vi "Autonomous Independent.vi"() -> ()   [LabVIEW 2014]
doc: "This VI is called when autonomous begins, and will automatically be terminated when autonomous ends. You can carry out timed or sensor driven robot movement independently without needing to return to the caller."
uses:
  <vilib>/Rock Robotics/WPI/Solenoid/WPI_SolenoidValue.ctl
  <vilib>/Rock Robotics/WPI/Joystick/WPI_JoystickGetSetRefNum.vi
  <vilib>/Rock Robotics/Network Tables/SD Write Numeric Array.vi
  <vilib>/Rock Robotics/Network Tables/SD Read Boolean.vi
  <vilib>/Rock Robotics/Network Tables/SD Write Boolean.vi
  <vilib>/Rock Robotics/WPI/RobotDrive/WPI_RobotDriveGetSetRefNum.vi
  <vilib>/Rock Robotics/WPI/RobotDrive/WPI_RobotDriveMecanumDrive_Cartesian.vi
  <vilib>/Rock Robotics/WPI/Solenoid/WPI_SolenoidSetEnum.vi
  <vilib>/Rock Robotics/Network Tables/SD Write String.vi
  Robot Global Data.vi
panel:
  out "Mode 3":bool
  out "error out":errorcluster
  out "Mode 1":bool
  out "Mode 0":bool
  in  "Turn":bool=TRUE
  in  "Lift":bool=TRUE
  in  "Move_Forward":bool=TRUE
  in  "Start":bool=TRUE
  in  "Begin":bool=TRUE
  in  "Lift_Time":dbl
  in  "Move_Foward_Time":dbl
  in  "Turn_Time":dbl
  in  "Start_Time":dbl
  # "Be sure to right-click and choose Data Operations>>Make Current Value default if you want to save the array values with the VI"
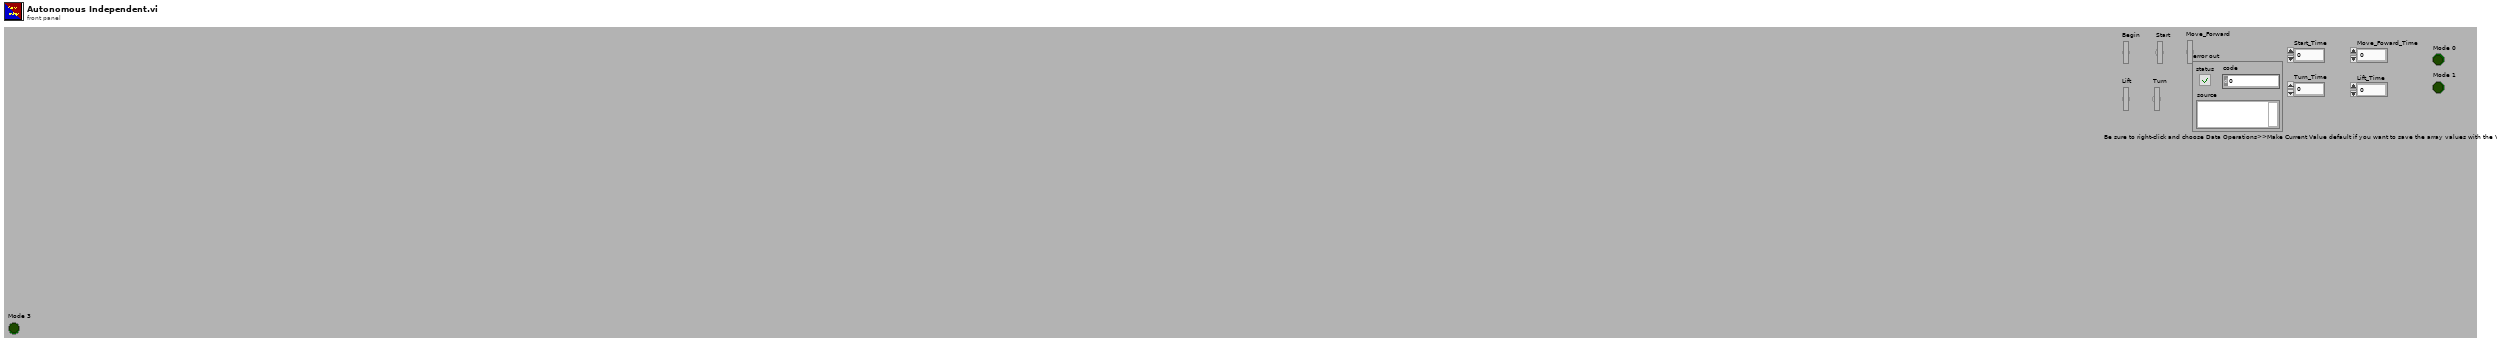
[diagram p1: front panel]
types:
  T1 = typedef "WPI_JoystickDevRef.ctl" = cluster{"Device":T2}
  T2 = typedef "WPI_JoystickDeviceEnum.ctl" = enum16{"USB 0", "USB 1", "USB 2", "USB 3", "USB 4", "USB 5"}
  T3 = typedef "WPI_SolenoidValue.ctl" = enum16{"Off", "On", "Forward", "Reverse"}
  T4 = typedef "WPI_MotorControlDeviceRef.ctl" = cluster{"DeviceStatus":errorcluster, "Type":T5, "PWM":cluster{"Controller":T6, "PWM Channel":T7, "DeadBand":T8}, "CAN":cluster{"Device Number":u8, "Control Mode":T9, "Semaphore":T10, "Max Vout":dbl, "TalonSRX Control Mode":T11}, "Invert":bool, "TransformRef":T12, "InvTransformRef":T12}
  T5 = typedef "WPI_MotorControlType.ctl" = enum16{"PWM", "CAN", "CANTalonSRX"}
  T6 = typedef "FPGA_TypedefDigitalModule.ctl" = enum16{"Controller 1"}
  T7 = typedef "FPGA_DIOPWMChannel.ctl" = enum8{"PWM 0", "PWM 1", "PWM 2", "PWM 3", "PWM 4", "PWM 5", "PWM 6", "PWM 7", "PWM 8", "PWM 9", "PWM MXP 0", "PWM MXP 1", "PWM MXP 2", "PWM MXP 3", "PWM MXP 4", "PWM MXP 5", "PWM MXP 6", "PWM MXP 7", "PWM MXP 8", "PWM MXP 9", "Invalid"}
  T8 = typedef "WPI_PWMDeadband.ctl" = cluster{"Name":string, "maxPositivePwm":i32, "minPositivePwm":i32, "centerPwm":i32, "maxNegativePwm":i32, "minNegativePwm":i32, "angularRange":u16}
  T9 = typedef "WPI_CANJaguar_ControlMode.ctl" = enum8{"Percent VBus", "Current", "Speed", "Position", "Voltage"}
  T10 = typedef "Semaphore RefNum" = refnum<k1>
  T11 = typedef "WPI_CANTalonSRX_APIControlMode.ctl" = enum8{"Percent VBus", "Speed", "Position", "Slave", "Unchanged / Invalid"}
  T12 = typedef "WPI_PWMTransform_ConPane.ctl" = refnum<vi>
  T13 = typedef "WPI_RobotDriveDevRef.ctl" = cluster{"DevStatus":errorcluster, "Motors[]":T4[], "Square Inputs":bool, "Max Output":dbl}
  T14 = typedef "WPI_ServoDeviceRef.ctl" = cluster{"DeviceStatus":errorcluster, "Controller":T6, "PWM Channel":T7, "DeadBand":T8}
  T15 = typedef "WPI_SolenoidDevRef.ctl" = cluster{"DevStatus":errorcluster, "Pneumatics Control Module":u8, "Forward Solenoid Channel":T16, "Reverse Solenoid Channel":T16}
  T16 = typedef "WPI_SolenoidChannel.ctl" = enum8{"Solenoid 0", "Solenoid 1", "Solenoid 2", "Solenoid 3", "Solenoid 4", "Solenoid 5", "Solenoid 6", "Solenoid 7", "Invalid"}
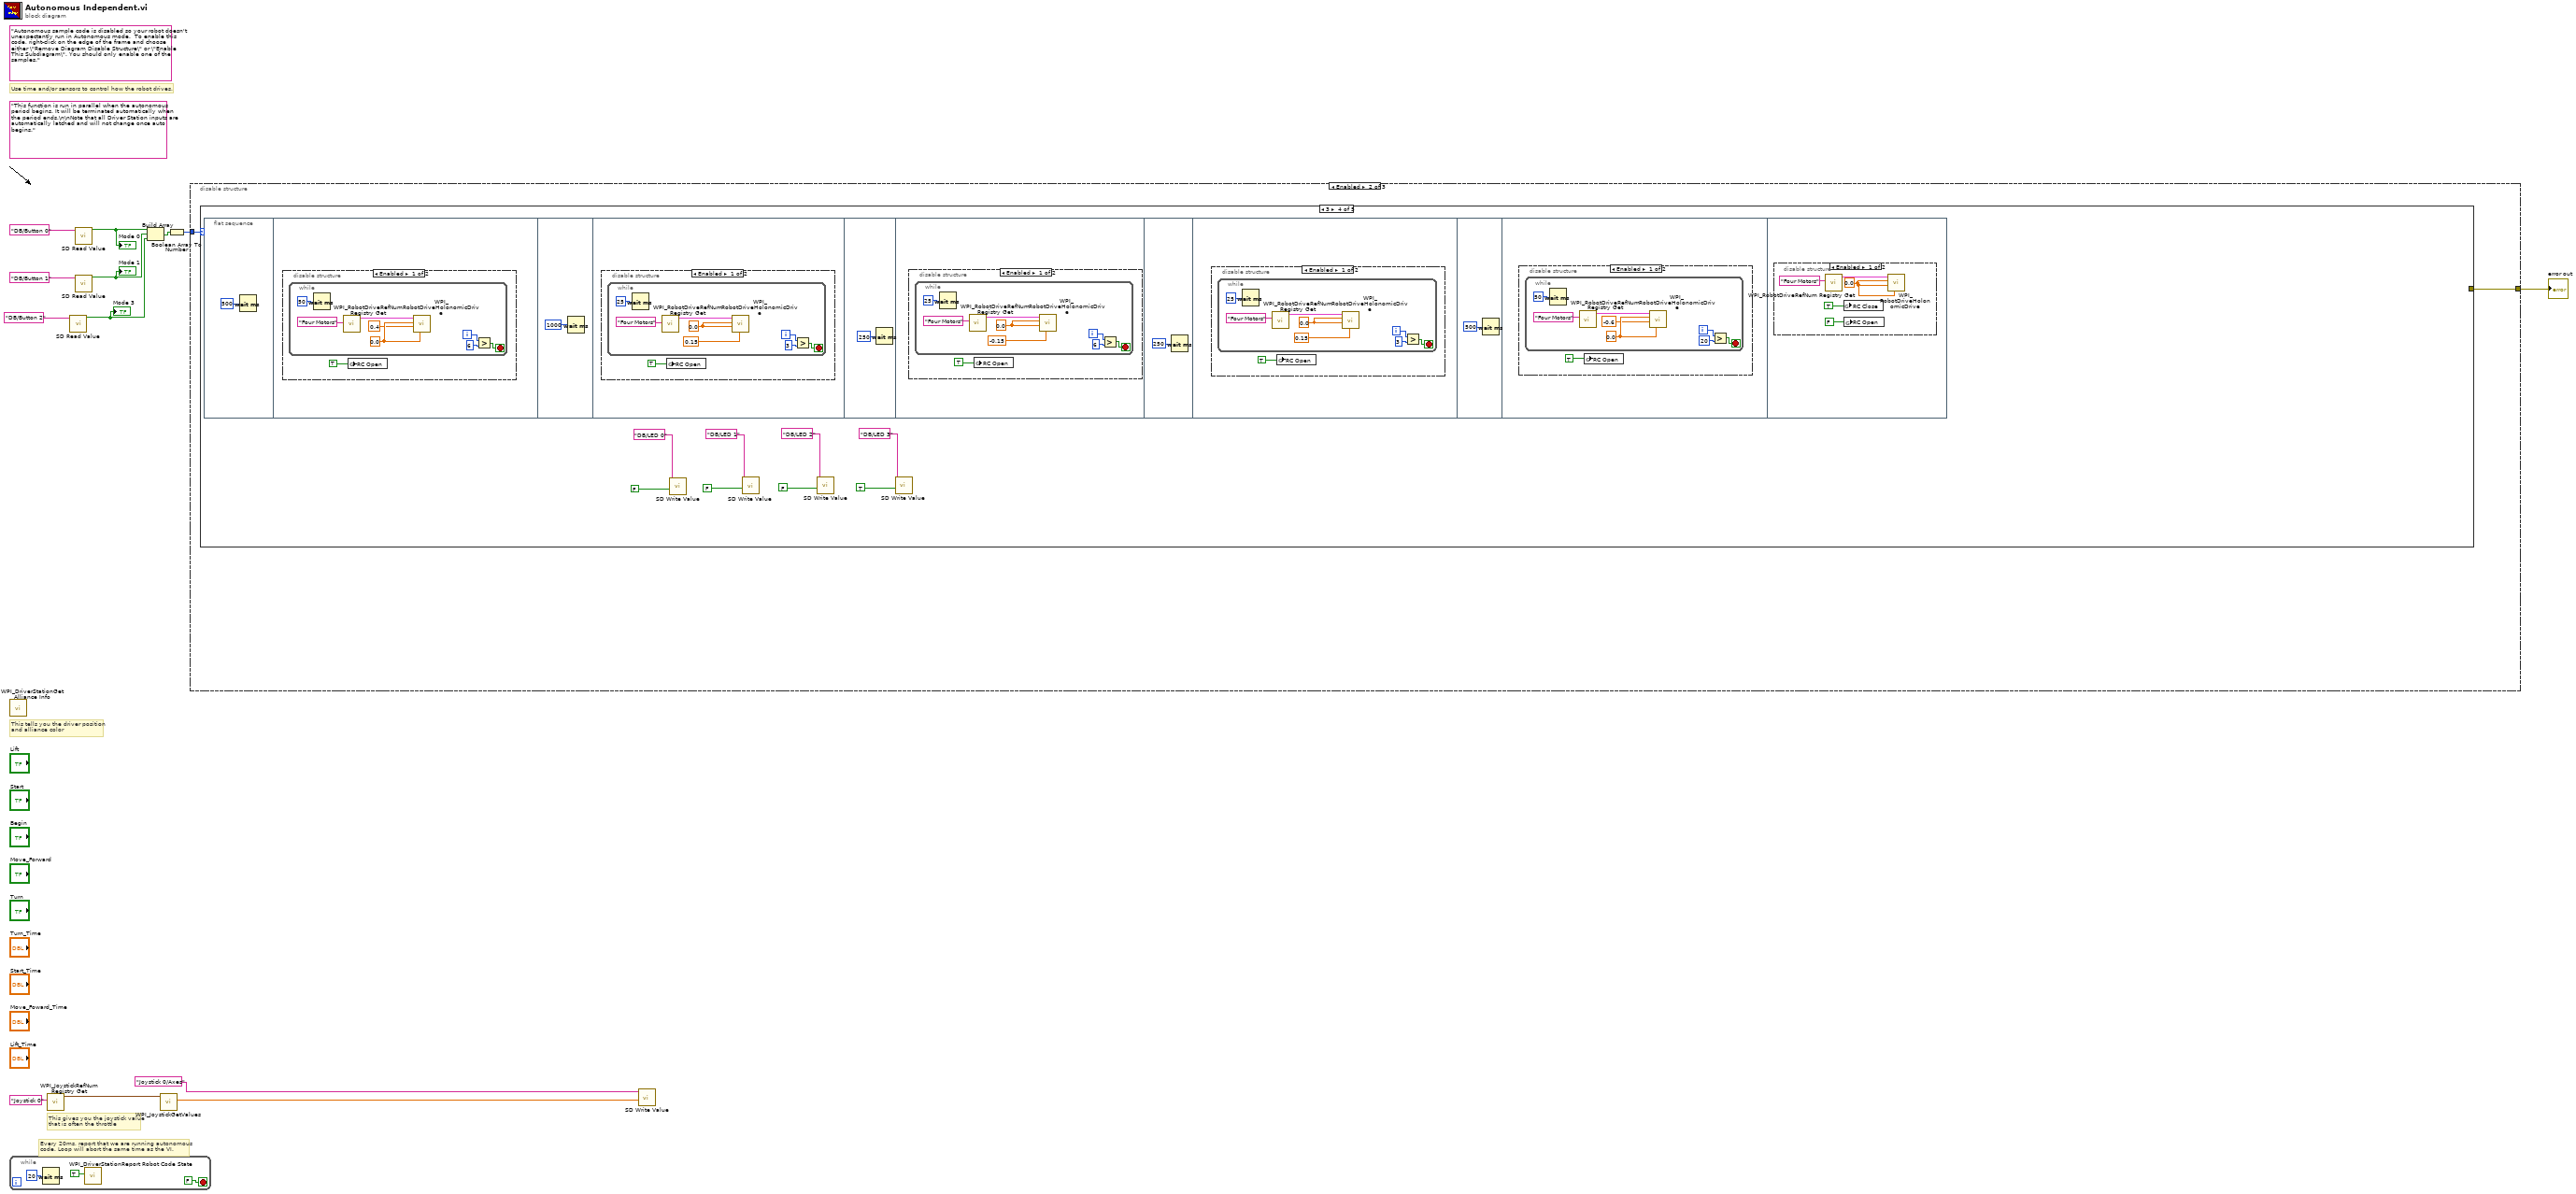
[diagram p0: block diagram]
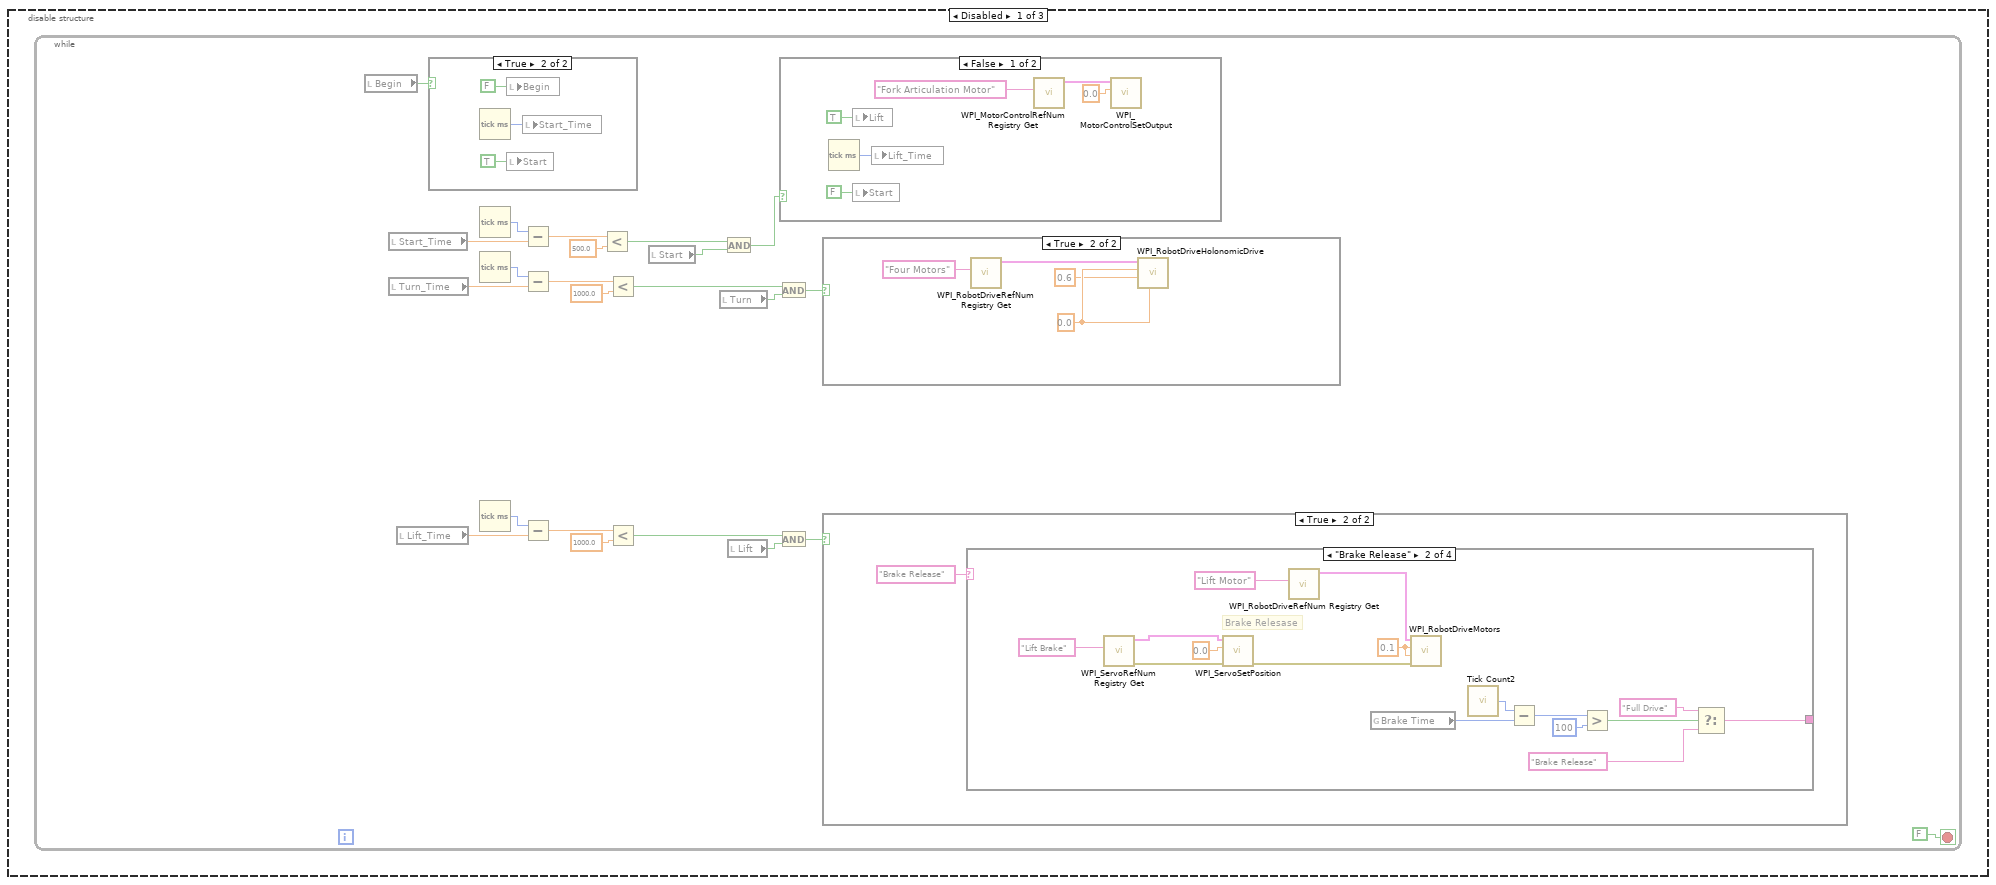
[diagram p2: hidden frame]
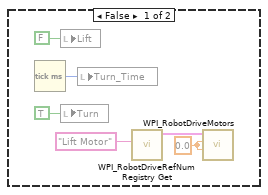
[diagram p3: hidden frame]
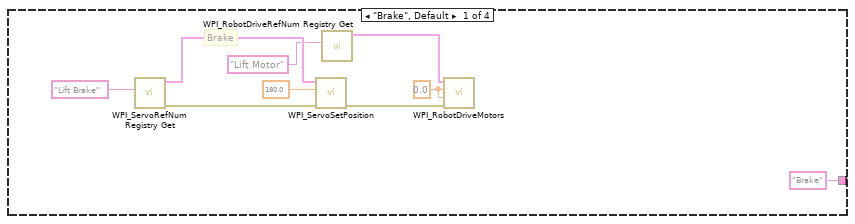
[diagram p4: hidden frame]
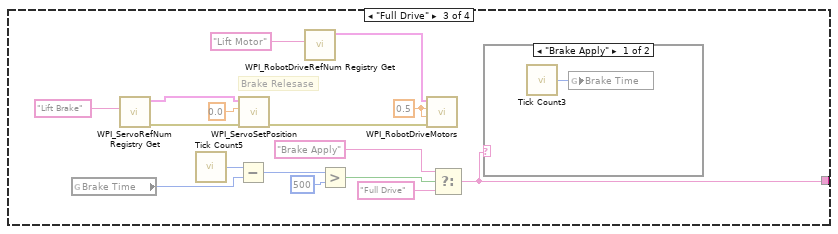
[diagram p5: hidden frame]
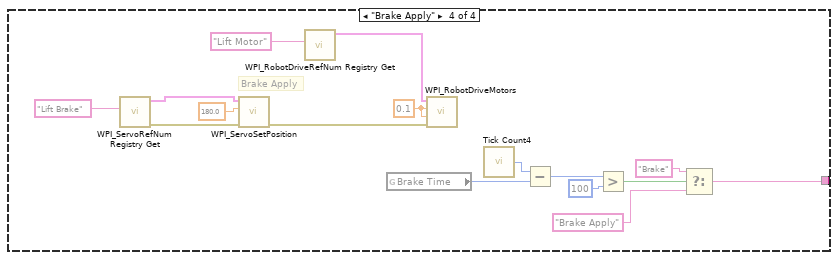
[diagram p7: hidden frame]
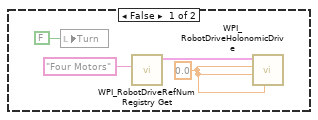
[diagram p8: hidden frame]
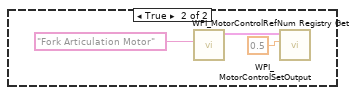
[diagram p9: hidden frame]
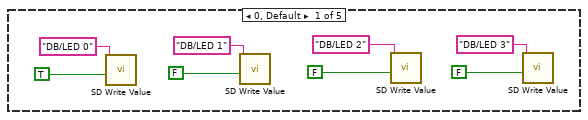
[diagram p11: hidden frame]
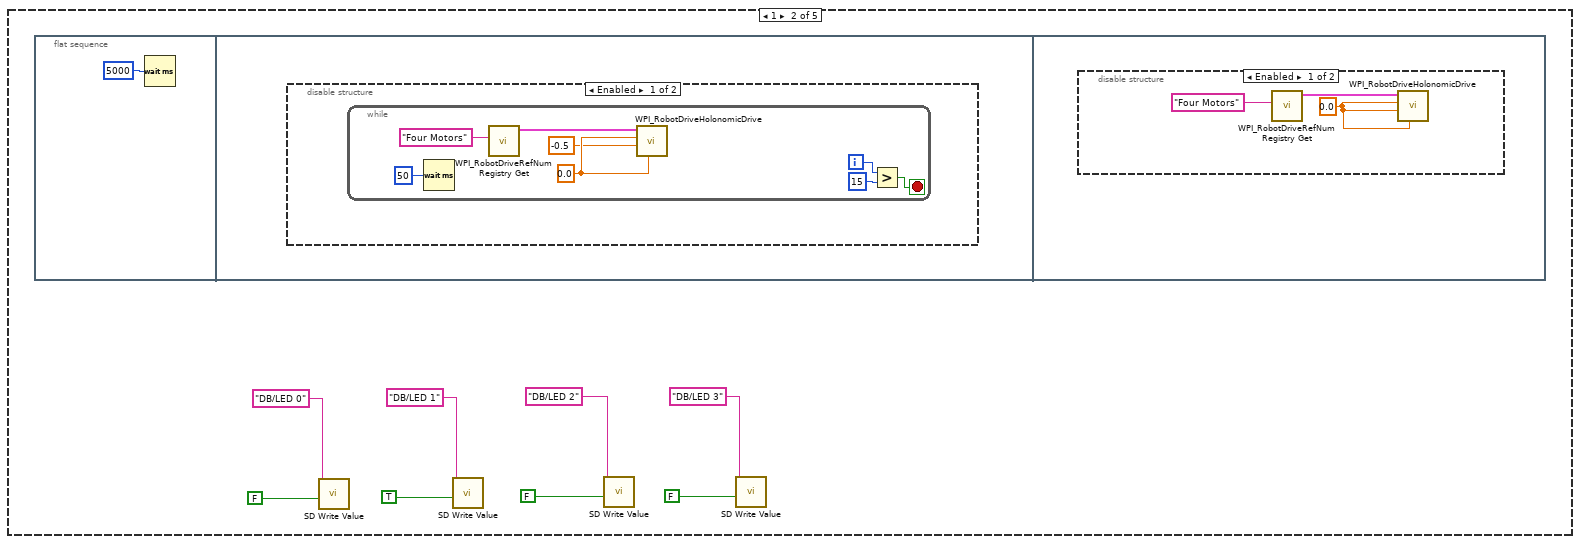
[diagram p12: hidden frame]
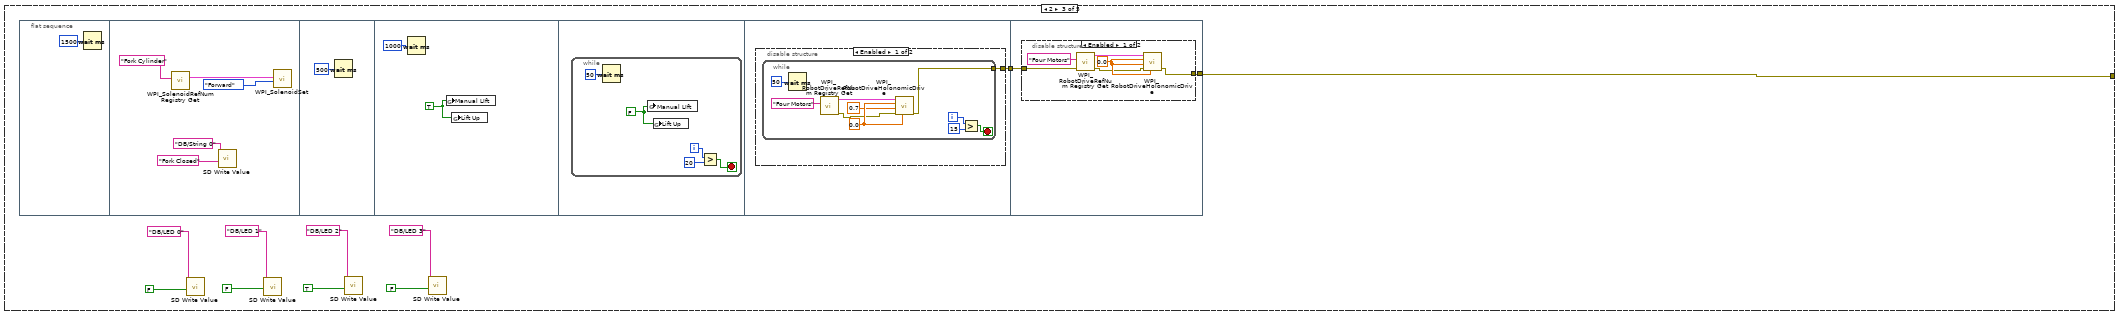
[diagram p15: hidden frame]
diagram:
  (unwired) "Autonomous sample code is disabled so your robot doesn't unexpectantly run in Autonomous mode.  To enable this code, right-click on the edge of the frame and choose either \"Remove Diagram Disable Structure\" or \"Enable This Subdiagram\". You should only enable one of the samples."
  (unwired) "This function is run in parallel when the autonomous period begins. It will be terminated automatically when the period ends.\n\nNote that all Driver Station inputs are automatically latched and will not change once auto begins."
  # "Every 20ms, report that we are running autonomous\ncode. Loop will abort the same time as the VI."
  # "This gives you the joystick value\nthat is often the throttle"
  # "Use time and/or sensors to control how the robot drives."
  # "This tells you the driver position\nand alliance color"
  n1 = call <vilib>:"WPI_DriverStationGet Alliance Info.vi"() -> ()  [unwired: 12 out]
  n2 = while {
    stop <- FALSE stop-if-true
    n3 = Wait (ms)(milliseconds to wait=u32 20) -> ()  [unwired: 1 out]
    n4 = call <vilib>:"WPI_DriverStationReport Robot Code State.vi"("Autonomous"=TRUE) -> ()  [unwired: 10 in, 1 out]
  }
  n5 = call <vilib>:"WPI_JoystickRefNum Registry Get.vi"("refnum name"="Joystick 0") -> ("JoystickDevRef"=w12:T1)  [unwired: 1 in, 9 out]
  n6 = call-poly <vilib>:"SD Read Value.vi"("Name"="DB/Button 2" ("refnum name")) -> ("Boolean"=w1:bool)  [unwired: 8 in, 2 out]
  "Mode 3" <- w1
  n7 = call-poly <vilib>:"SD Read Value.vi"("Name"="DB/Button 0" ("refnum name")) -> ("Boolean"=w7:bool)  [unwired: 8 in, 2 out]
  "Mode 0" <- w7
  n8 = call-poly <vilib>:"SD Read Value.vi"("Name"="DB/Button 1" ("refnum name")) -> ("Boolean"=w6:bool)  [unwired: 8 in, 2 out]
  "Mode 1" <- w6
  n9 = Build Array(w7, w6, w1) -> (w5:bool[])
  n10 = call <vilib>:"WPI_JoystickGetValues.vi"("JoystickDevRef"=w12) -> ("Axes"=w10:dbl[])  [unwired: 6 in, 4 out]
  n11 = Boolean Array To Number(Boolean array=w5) -> (number=w4:u32)
  n12 = disable-structure shown="Enabled" {
    disable-tunnel: w4 -> [_ w126 _]
    disable-tunnel: [_ w125 _] -> w3
    frame Disabled {
      n13 = while {
        stop <- FALSE stop-if-true
        n14 = local read "Begin"() -> (w20:bool)
        n15 = local read "Start_Time"() -> (w37:dbl)
        n16 = local read "Turn_Time"() -> (w31:dbl)
        n17 = local read "Lift_Time"() -> (w22:dbl)
        n18 = case shown="True" w20 {
          frame False {
          }
          frame True {
            n19 = Tick Count (ms)() -> (millisecond timer value=w124:u32)
            n20 = local write "Begin"(FALSE ("Begin")) -> ()
            n21 = local write "Start"(TRUE ("Start")) -> ()
            n22 = local write "Start_Time"(w124) -> ()
          }
        }
        n23 = Tick Count (ms)() -> (millisecond timer value=w38:u32)
        n24 = Tick Count (ms)() -> (millisecond timer value=w32:u32)
        n25 = Tick Count (ms)() -> (millisecond timer value=w23:u32)
        n26 = Subtract(x=w38, y=w37) -> (x-y=w36:dbl)
        n27 = Subtract(x=w32, y=w31) -> (x-y=w28:dbl)
        n28 = Subtract(x=w23, y=w22) -> (x-y=w24:dbl)
        n29 = Less?(x=w36, y=500.0) -> (x < y?=w34:bool)
        n30 = Less?(x=w28, y=1000.0) -> (x < y?=w29:bool)
        n31 = Less?(x=w24, y=1000.0) -> (x < y?=w25:bool)
        n32 = local read "Start"() -> (w18:bool)
        n33 = local read "Turn"() -> (w17:bool)
        n34 = And(x=w34, y=w18) -> (x .and. y?=w33:bool)
        n35 = local read "Lift"() -> (w19:bool)
        n36 = And(x=w29, y=w17) -> (x .and. y?=w27:bool)
        n37 = And(x=w25, y=w19) -> (x .and. y?=w21:bool)
        n38 = case shown="False" w33 {
          frame False {
            n39 = Tick Count (ms)() -> (millisecond timer value=w115:u32)
            n40 = local write "Lift"(TRUE ("Lift")) -> ()
            n41 = local write "Start"(FALSE ("Start")) -> ()
            n42 = local write "Lift_Time"(w115) -> ()
            n43 = call <vilib>:"WPI_MotorControlRefNum Registry Get.vi"("refnum name"="Fork Articulation Motor") -> ("MotorControlDevRef"=w116:T4)  [unwired: 9 in, 1 out]
            n44 = call <vilib>:"WPI_MotorControlSetOutput.vi"("Output"=0.0, "MotorControlDevRef"=w116) -> ()  [unwired: 7 in, 3 out]
          }
          frame True {
            n45 = call <vilib>:"WPI_MotorControlRefNum Registry Get.vi"("refnum name"="Fork Articulation Motor") -> ("MotorControlDevRef"=w119:T4)  [unwired: 9 in, 1 out]
            n46 = call <vilib>:"WPI_MotorControlSetOutput.vi"("Output"=0.5, "MotorControlDevRef"=w119) -> ()  [unwired: 7 in, 3 out]
          }
        }
        n47 = case shown="True" w27 {
          frame False {
            w106 = 0.0 ("Rotation")
            n48 = local write "Turn"(FALSE ("Turn")) -> ()
            n49 = call <vilib>:"WPI_RobotDriveRefNum Registry Get.vi"("refnum name"="Four Motors") -> ("RobotDriveDevRef"=w107:T13)  [unwired: 1 in, 9 out]
            n50 = call-poly <vilib>:"WPI_RobotDriveHolonomicDrive.vi"("Rotation"=w106, "Y"=w106, "X"=w106, "RobotDriveDevRef"=w107) -> ()  [unwired: 5 in, 3 out]
          }
          frame True {
            w110 = 0.0 ("Rotation")
            n51 = call <vilib>:"WPI_RobotDriveRefNum Registry Get.vi"("refnum name"="Four Motors") -> ("RobotDriveDevRef"=w111:T13)  [unwired: 1 in, 9 out]
            n52 = call-poly <vilib>:"WPI_RobotDriveHolonomicDrive.vi"("Rotation"=w110, "Y"=0.6, "X"=w110, "RobotDriveDevRef"=w111) -> ()  [unwired: 5 in, 3 out]
          }
        }
        n53 = case shown="True" w21 {
          frame False {
            w42 = 0.0 ("RightSpeed")
            n54 = Tick Count (ms)() -> (millisecond timer value=w45:u32)
            n55 = local write "Lift"(FALSE ("Lift")) -> ()
            n56 = local write "Turn"(TRUE ("Turn")) -> ()
            n57 = local write "Turn_Time"(w45) -> ()
            n58 = call <vilib>:"WPI_RobotDriveRefNum Registry Get.vi"("refnum name"="Lift Motor") -> ("RobotDriveDevRef"=w43:T13)  [unwired: 9 in, 1 out]
            n59 = call <vilib>:"WPI_RobotDriveMotors.vi"("RightSpeed"=w42, "LeftSpeed"=w42, "RobotDriveDevRef"=w43) -> ()  [unwired: 6 in, 3 out]
          }
          frame True {
            n60 = case shown="\"Brake Release\"" "Brake Release" {
              tunnel: ["Brake" w56 w80 w89] -> _
              frame "Brake", Default {
                w50 = 0.0 ("LeftSpeed")
                # "Brake"
                n61 = call <vilib>:"WPI_ServoRefNum Registry Get.vi"("refnum name"="Lift Brake") -> ("error out"=w48:errorcluster, "ServoDeviceRef"=w53:T14)  [unwired: 9 in]
                n62 = call <vilib>:"WPI_ServoSetPosition.vi"("error in (no error)"=w48, "Position"=180.0, "ServoDeviceRef"=w53) -> ("error out"=w49:errorcluster)  [unwired: 7 in, 1 out]
                n63 = call <vilib>:"WPI_RobotDriveRefNum Registry Get.vi"("refnum name"="Lift Motor") -> ("RobotDriveDevRef"=w51:T13)  [unwired: 9 in, 1 out]
                n64 = call <vilib>:"WPI_RobotDriveMotors.vi"("error in (no error)"=w49, "RightSpeed"=w50, "LeftSpeed"=w50, "RobotDriveDevRef"=w51) -> ()  [unwired: 5 in, 3 out]
              }
              frame "Brake Release" {
                w64 = 0.1 ("RightSpeed")
                # "Brake Relesase"
                n65 = call <vilib>:"WPI_ServoRefNum Registry Get.vi"("refnum name"="Lift Brake") -> ("error out"=w66:errorcluster, "ServoDeviceRef"=w69:T14)  [unwired: 9 in]
                n66 = call <vilib>:"WPI_ServoSetPosition.vi"("error in (no error)"=w66, "Position"=0.0, "ServoDeviceRef"=w69) -> ("error out"=w65:errorcluster)  [unwired: 7 in, 1 out]
                n67 = call <vilib>:"WPI_RobotDriveRefNum Registry Get.vi"("refnum name"="Lift Motor") -> ("RobotDriveDevRef"=w67:T13)  [unwired: 9 in, 1 out]
                n68 = global read "Robot Global Data.vi" "Brake Time"() -> (w57:u32)
                n69 = call <vilib>:"WPI_RobotDriveMotors.vi"("error in (no error)"=w65, "RightSpeed"=w64, "LeftSpeed"=w64, "RobotDriveDevRef"=w67) -> ()  [unwired: 5 in, 3 out]
                n70 = call "Tick Count2"() -> ("Tick Count(mSec)"=w58:u32)
                n71 = Subtract(x=w58, y=w57) -> (x-y=w61:u32)
                n72 = Greater?(x=w61, y=u32 100) -> (0:w62:bool)
                n73 = Select(t="Full Drive", s=w62, f="Brake Release") -> (s? t:f=w56:string)
              }
              frame "Full Drive" {
                w79 = 0.5 ("RightSpeed")
                # "Brake Relesase"
                n74 = global read "Robot Global Data.vi" "Brake Time"() -> (w78:u32)
                n75 = call <vilib>:"WPI_ServoRefNum Registry Get.vi"("refnum name"="Lift Brake") -> ("error out"=w82:errorcluster, "ServoDeviceRef"=w85:T14)  [unwired: 9 in]
                n76 = call "Tick Count5"() -> ("Tick Count(mSec)"=w77:u32)
                n77 = Subtract(x=w77, y=w78) -> (x-y=w75:u32)
                n78 = call <vilib>:"WPI_ServoSetPosition.vi"("error in (no error)"=w82, "Position"=0.0, "ServoDeviceRef"=w85) -> ("error out"=w81:errorcluster)  [unwired: 7 in, 1 out]
                n79 = call <vilib>:"WPI_RobotDriveRefNum Registry Get.vi"("refnum name"="Lift Motor") -> ("RobotDriveDevRef"=w83:T13)  [unwired: 9 in, 1 out]
                n80 = Greater?(x=w75, y=u32 500) -> (0:w72:bool)
                n81 = call <vilib>:"WPI_RobotDriveMotors.vi"("error in (no error)"=w81, "RightSpeed"=w79, "LeftSpeed"=w79, "RobotDriveDevRef"=w83) -> ()  [unwired: 5 in, 3 out]
                n82 = Select(t="Brake Apply", s=w72, f="Full Drive") -> (s? t:f=w80:string)
                n83 = case shown="\"Brake Apply\"" w80 {
                  frame "Brake Apply" {
                    n84 = call "Tick Count3"() -> ("Tick Count(mSec)"=w88:u32)
                    n85 = global write "Robot Global Data.vi" "Brake Time"(w88) -> ()
                  }
                  frame "Full Drive", Default {
                  }
                }
              }
              frame "Brake Apply" {
                w104 = 0.1 ("RightSpeed")
                # "Brake Apply"
                n86 = call <vilib>:"WPI_ServoRefNum Registry Get.vi"("refnum name"="Lift Brake") -> ("error out"=w102:errorcluster, "ServoDeviceRef"=w99:T14)  [unwired: 9 in]
                n87 = call <vilib>:"WPI_ServoSetPosition.vi"("error in (no error)"=w102, "Position"=180.0, "ServoDeviceRef"=w99) -> ("error out"=w103:errorcluster)  [unwired: 7 in, 1 out]
                n88 = call <vilib>:"WPI_RobotDriveRefNum Registry Get.vi"("refnum name"="Lift Motor") -> ("RobotDriveDevRef"=w101:T13)  [unwired: 9 in, 1 out]
                n89 = global read "Robot Global Data.vi" "Brake Time"() -> (w91:u32)
                n90 = call <vilib>:"WPI_RobotDriveMotors.vi"("error in (no error)"=w103, "RightSpeed"=w104, "LeftSpeed"=w104, "RobotDriveDevRef"=w101) -> ()  [unwired: 5 in, 3 out]
                n91 = call "Tick Count4"() -> ("Tick Count(mSec)"=w92:u32)
                n92 = Subtract(x=w92, y=w91) -> (x-y=w90:u32)
                n93 = Greater?(x=w90, y=u32 100) -> (0:w93:bool)
                n94 = Select(t="Brake", s=w93, f="Brake Apply") -> (s? t:f=w89:string)
              }
            }
          }
        }
      }
    }
    frame Enabled {
      n95 = case shown="3" w126 {
        tunnel: [_ _ w155 _ _] -> w125
        frame 0, Default {
          n96 = call-poly <vilib>:"SD Write Value.vi"("Boolean"=TRUE, "Name"="DB/LED 0") -> ()  [unwired: 8 in, 2 out]
          n97 = call-poly <vilib>:"SD Write Value.vi"("Boolean"=FALSE, "Name"="DB/LED 1") -> ()  [unwired: 8 in, 2 out]
          n98 = call-poly <vilib>:"SD Write Value.vi"("Boolean"=FALSE, "Name"="DB/LED 2") -> ()  [unwired: 8 in, 2 out]
          n99 = call-poly <vilib>:"SD Write Value.vi"("Boolean"=FALSE, "Name"="DB/LED 3") -> ()  [unwired: 8 in, 2 out]
        }
        frame 1 {
          n100 = flat-sequence {
            frame #0 {
              n101 = Wait (ms)(milliseconds to wait=u32 5000) -> ()  [unwired: 1 out]
            }
            frame #1 {
              n102 = disable-structure shown="Enabled" {
                frame Enabled {
                  n103 = while {
                    i -> [w148]
                    stop <- w146 stop-if-true
                    w145 = 0.0 ("Rotation")
                    n104 = Wait (ms)(milliseconds to wait=u32 50) -> ()  [unwired: 1 out]
                    n105 = call <vilib>:"WPI_RobotDriveRefNum Registry Get.vi"("refnum name"="Four Motors") -> ("RobotDriveDevRef"=w151:T13)  [unwired: 1 in, 9 out]
                    n106 = call-poly <vilib>:"WPI_RobotDriveHolonomicDrive.vi"("Rotation"=w145, "Y"=-0.5, "X"=w145, "RobotDriveDevRef"=w151) -> ()  [unwired: 5 in, 3 out]
                    n107 = Greater?(x=w148, y=15) -> (0:w146:bool)
                  }
                }
                frame Disabled {
                }
              }
            }
            frame #2 {
              n108 = disable-structure shown="Enabled" {
                frame Enabled {
                  w152 = 0.0 ("Rotation")
                  n109 = call <vilib>:"WPI_RobotDriveRefNum Registry Get.vi"("refnum name"="Four Motors") -> ("RobotDriveDevRef"=w154:T13)  [unwired: 1 in, 9 out]
                  n110 = call-poly <vilib>:"WPI_RobotDriveHolonomicDrive.vi"("Rotation"=w152, "Y"=w152, "X"=w152, "RobotDriveDevRef"=w154) -> ()  [unwired: 5 in, 3 out]
                }
                frame Disabled {
                }
              }
            }
          }
          n111 = call-poly <vilib>:"SD Write Value.vi"("Boolean"=FALSE, "Name"="DB/LED 0") -> ()  [unwired: 8 in, 2 out]
          n112 = call-poly <vilib>:"SD Write Value.vi"("Boolean"=TRUE, "Name"="DB/LED 1") -> ()  [unwired: 8 in, 2 out]
          n113 = call-poly <vilib>:"SD Write Value.vi"("Boolean"=FALSE, "Name"="DB/LED 2") -> ()  [unwired: 8 in, 2 out]
          n114 = call-poly <vilib>:"SD Write Value.vi"("Boolean"=FALSE, "Name"="DB/LED 3") -> ()  [unwired: 8 in, 2 out]
        }
        frame 2 {
          n115 = flat-sequence {
            tunnel: [w179] -> w156
            tunnel: w156 -> [w193]
            tunnel: [w192] -> w155
            frame #0 {
              n116 = Wait (ms)(milliseconds to wait=u32 1500) -> ()  [unwired: 1 out]
            }
            frame #1 {
              n117 = call <vilib>:"WPI_SolenoidRefNum Registry Get.vi"("refnum name"="Fork Cylinder") -> ("SolenoidDevRef"=w170:T15)  [unwired: 9 in, 1 out]
              n118 = call-poly <vilib>:"SD Write Value.vi"("String"="Fork Closed", "Name"="DB/String 0") -> ()  [unwired: 8 in, 2 out]
              n119 = call-poly <vilib>:"WPI_SolenoidSet.vi"("Value"=WPI_SolenoidValue."Forward", "SolenoidDevRef"=w170) -> ()  [unwired: 1 in, 9 out]
            }
            frame #2 {
              n120 = Wait (ms)(milliseconds to wait=u32 500) -> ()  [unwired: 1 out]
            }
            frame #3 {
              w173 = TRUE
              n121 = Wait (ms)(milliseconds to wait=u32 1000) -> ()  [unwired: 1 out]
              n122 = global write "Robot Global Data.vi" "Manual LIft"(w173) -> ()
              n123 = global write "Robot Global Data.vi" "Lift Up"(w173) -> ()
            }
            frame #4 {
              n124 = while {
                i -> [w175]
                stop <- w176 stop-if-true
                w178 = FALSE
                n125 = Wait (ms)(milliseconds to wait=u32 50) -> ()  [unwired: 1 out]
                n126 = global write "Robot Global Data.vi" "Manual LIft"(w178) -> ()
                n127 = global write "Robot Global Data.vi" "Lift Up"(w178) -> ()
                n128 = Greater?(x=w175, y=20) -> (0:w176:bool)
              }
            }
            frame #5 {
              n129 = disable-structure shown="Enabled" {
                disable-tunnel: [w180 w191] -> w179
                frame Enabled {
                  n130 = while {
                    tunnel: [w181] -> w180
                    i -> [w187]
                    stop <- w185 stop-if-true
                    w184 = 0.0 ("Rotation")
                    n131 = Wait (ms)(milliseconds to wait=u32 50) -> ()  [unwired: 1 out]
                    n132 = call <vilib>:"WPI_RobotDriveRefNum Registry Get.vi"("refnum name"="Four Motors") -> ("error out"=w182:errorcluster, "RobotDriveDevRef"=w190:T13)  [unwired: 1 in, 8 out]
                    n133 = call-poly <vilib>:"WPI_RobotDriveHolonomicDrive.vi"("Rotation"=w184, "error in (no error)"=w182, "Y"=0.7, "X"=w184, "RobotDriveDevRef"=w190) -> ("error out"=w181:errorcluster)  [unwired: 4 in, 2 out]
                    n134 = Greater?(x=w187, y=15) -> (0:w185:bool)
                  }
                }
                frame Disabled {
                }
              }
            }
            frame #6 {
              n135 = disable-structure shown="Enabled" {
                disable-tunnel: w193 -> [w196 w200]
                disable-tunnel: [w194 w200] -> w192
                frame Enabled {
                  w197 = 0.0 ("Rotation")
                  n136 = call <vilib>:"WPI_RobotDriveRefNum Registry Get.vi"("error in (no error)"=w196, "refnum name"="Four Motors") -> ("error out"=w195:errorcluster, "RobotDriveDevRef"=w199:T13)  [unwired: 8 out]
                  n137 = call-poly <vilib>:"WPI_RobotDriveHolonomicDrive.vi"("Rotation"=w197, "error in (no error)"=w195, "Y"=w197, "X"=w197, "RobotDriveDevRef"=w199) -> ("error out"=w194:errorcluster)  [unwired: 4 in, 2 out]
                }
                frame Disabled {
                }
              }
            }
          }
          n138 = call-poly <vilib>:"SD Write Value.vi"("Boolean"=FALSE, "Name"="DB/LED 0") -> ()  [unwired: 8 in, 2 out]
          n139 = call-poly <vilib>:"SD Write Value.vi"("Boolean"=FALSE, "Name"="DB/LED 1") -> ()  [unwired: 8 in, 2 out]
          n140 = call-poly <vilib>:"SD Write Value.vi"("Boolean"=TRUE, "Name"="DB/LED 2") -> ()  [unwired: 8 in, 2 out]
          n141 = call-poly <vilib>:"SD Write Value.vi"("Boolean"=FALSE, "Name"="DB/LED 3") -> ()  [unwired: 8 in, 2 out]
        }
        frame 3 {
          n142 = flat-sequence {
            frame #0 {
              n143 = Wait (ms)(milliseconds to wait=u32 500) -> ()  [unwired: 1 out]
            }
            frame #1 {
              n144 = disable-structure shown="Enabled" {
                frame Enabled {
                  n145 = while {
                    i -> [w215]
                    stop <- w213 stop-if-true
                    w212 = 0.0 ("Rotation")
                    n146 = Wait (ms)(milliseconds to wait=u32 50) -> ()  [unwired: 1 out]
                    n147 = call <vilib>:"WPI_RobotDriveRefNum Registry Get.vi"("refnum name"="Four Motors") -> ("RobotDriveDevRef"=w218:T13)  [unwired: 1 in, 9 out]
                    n148 = call-poly <vilib>:"WPI_RobotDriveHolonomicDrive.vi"("Rotation"=w212, "Y"=0.4, "X"=w212, "RobotDriveDevRef"=w218) -> ()  [unwired: 5 in, 3 out]
                    n149 = Greater?(x=w215, y=6) -> (0:w213:bool)
                  }
                  n150 = global write "Robot Global Data.vi" "RC Open"(TRUE ("Enable Vision")) -> ()
                }
                frame Disabled {
                }
              }
            }
            frame #2 {
              n151 = Wait (ms)(milliseconds to wait=u32 1000) -> ()  [unwired: 1 out]
            }
            frame #3 {
              n152 = disable-structure shown="Enabled" {
                frame Enabled {
                  n153 = while {
                    i -> [w225]
                    stop <- w223 stop-if-true
                    w221 = 0.0 ("Y")
                    n154 = Wait (ms)(milliseconds to wait=u32 25) -> ()  [unwired: 1 out]
                    n155 = call <vilib>:"WPI_RobotDriveRefNum Registry Get.vi"("refnum name"="Four Motors") -> ("RobotDriveDevRef"=w228:T13)  [unwired: 1 in, 9 out]
                    n156 = call-poly <vilib>:"WPI_RobotDriveHolonomicDrive.vi"("Rotation"=0.15, "Y"=w221, "X"=w221, "RobotDriveDevRef"=w228) -> ()  [unwired: 5 in, 3 out]
                    n157 = Greater?(x=w225, y=3) -> (0:w223:bool)
                  }
                  n158 = global write "Robot Global Data.vi" "RC Open"(TRUE ("Enable Vision")) -> ()
                }
                frame Disabled {
                }
              }
            }
            frame #4 {
              n159 = Wait (ms)(milliseconds to wait=u32 250) -> ()  [unwired: 1 out]
            }
            frame #5 {
              n160 = disable-structure shown="Enabled" {
                frame Enabled {
                  n161 = while {
                    i -> [w235]
                    stop <- w233 stop-if-true
                    w231 = 0.0 ("Y")
                    n162 = Wait (ms)(milliseconds to wait=u32 25) -> ()  [unwired: 1 out]
                    n163 = call <vilib>:"WPI_RobotDriveRefNum Registry Get.vi"("refnum name"="Four Motors") -> ("RobotDriveDevRef"=w238:T13)  [unwired: 1 in, 9 out]
                    n164 = call-poly <vilib>:"WPI_RobotDriveHolonomicDrive.vi"("Rotation"=-0.15, "Y"=w231, "X"=w231, "RobotDriveDevRef"=w238) -> ()  [unwired: 5 in, 3 out]
                    n165 = Greater?(x=w235, y=6) -> (0:w233:bool)
                  }
                  n166 = global write "Robot Global Data.vi" "RC Open"(TRUE ("Enable Vision")) -> ()
                }
                frame Disabled {
                }
              }
            }
            frame #6 {
              n167 = Wait (ms)(milliseconds to wait=u32 250) -> ()  [unwired: 1 out]
            }
            frame #7 {
              n168 = disable-structure shown="Enabled" {
                frame Enabled {
                  n169 = while {
                    i -> [w245]
                    stop <- w243 stop-if-true
                    w241 = 0.0 ("Y")
                    n170 = Wait (ms)(milliseconds to wait=u32 25) -> ()  [unwired: 1 out]
                    n171 = call <vilib>:"WPI_RobotDriveRefNum Registry Get.vi"("refnum name"="Four Motors") -> ("RobotDriveDevRef"=w248:T13)  [unwired: 1 in, 9 out]
                    n172 = call-poly <vilib>:"WPI_RobotDriveHolonomicDrive.vi"("Rotation"=0.15, "Y"=w241, "X"=w241, "RobotDriveDevRef"=w248) -> ()  [unwired: 5 in, 3 out]
                    n173 = Greater?(x=w245, y=3) -> (0:w243:bool)
                  }
                  n174 = global write "Robot Global Data.vi" "RC Open"(TRUE ("Enable Vision")) -> ()
                }
                frame Disabled {
                }
              }
            }
            frame #8 {
              n175 = Wait (ms)(milliseconds to wait=u32 500) -> ()  [unwired: 1 out]
            }
            frame #9 {
              n176 = disable-structure shown="Enabled" {
                frame Enabled {
                  n177 = while {
                    i -> [w255]
                    stop <- w253 stop-if-true
                    w252 = 0.0 ("Rotation")
                    n178 = Wait (ms)(milliseconds to wait=u32 50) -> ()  [unwired: 1 out]
                    n179 = call <vilib>:"WPI_RobotDriveRefNum Registry Get.vi"("refnum name"="Four Motors") -> ("RobotDriveDevRef"=w258:T13)  [unwired: 1 in, 9 out]
                    n180 = call-poly <vilib>:"WPI_RobotDriveHolonomicDrive.vi"("Rotation"=w252, "Y"=-0.6, "X"=w252, "RobotDriveDevRef"=w258) -> ()  [unwired: 5 in, 3 out]
                    n181 = Greater?(x=w255, y=20) -> (0:w253:bool)
                  }
                  n182 = global write "Robot Global Data.vi" "RC Open"(TRUE ("Enable Vision")) -> ()
                }
                frame Disabled {
                }
              }
            }
            frame #10 {
              n183 = disable-structure shown="Enabled" {
                frame Enabled {
                  w261 = 0.0 ("Rotation")
                  n184 = call <vilib>:"WPI_RobotDriveRefNum Registry Get.vi"("refnum name"="Four Motors") -> ("RobotDriveDevRef"=w263:T13)  [unwired: 1 in, 9 out]
                  n185 = global write "Robot Global Data.vi" "RC Close"(TRUE ("Enable Vision")) -> ()
                  n186 = global write "Robot Global Data.vi" "RC Open"(FALSE ("Enable Vision")) -> ()
                  n187 = call-poly <vilib>:"WPI_RobotDriveHolonomicDrive.vi"("Rotation"=w261, "Y"=w261, "X"=w261, "RobotDriveDevRef"=w263) -> ()  [unwired: 5 in, 3 out]
                }
                frame Disabled {
                }
              }
            }
          }
          n188 = call-poly <vilib>:"SD Write Value.vi"("Boolean"=FALSE, "Name"="DB/LED 0") -> ()  [unwired: 8 in, 2 out]
          n189 = call-poly <vilib>:"SD Write Value.vi"("Boolean"=FALSE, "Name"="DB/LED 1") -> ()  [unwired: 8 in, 2 out]
          n190 = call-poly <vilib>:"SD Write Value.vi"("Boolean"=FALSE, "Name"="DB/LED 2") -> ()  [unwired: 8 in, 2 out]
          n191 = call-poly <vilib>:"SD Write Value.vi"("Boolean"=TRUE, "Name"="DB/LED 3") -> ()  [unwired: 8 in, 2 out]
        }
        frame 4 {
          n192 = flat-sequence {
            frame #0 {
              n193 = Wait (ms)(milliseconds to wait=u32 50) -> ()  [unwired: 1 out]
            }
            frame #1 {
              n194 = disable-structure shown="Enabled" {
                frame Enabled {
                  n195 = while {
                    i -> [w270]
                    stop <- w268 stop-if-true
                    w267 = 0.0 ("Rotation")
                    n196 = Wait (ms)(milliseconds to wait=u32 50) -> ()  [unwired: 1 out]
                    n197 = call <vilib>:"WPI_RobotDriveRefNum Registry Get.vi"("refnum name"="Four Motors") -> ("RobotDriveDevRef"=w273:T13)  [unwired: 1 in, 9 out]
                    n198 = call-poly <vilib>:"WPI_RobotDriveHolonomicDrive.vi"("Rotation"=w267, "Y"=0.3, "X"=w267, "RobotDriveDevRef"=w273) -> ()  [unwired: 5 in, 3 out]
                    n199 = Greater?(x=w270, y=4) -> (0:w268:bool)
                  }
                  n200 = global write "Robot Global Data.vi" "RC Open"(TRUE ("Enable Vision")) -> ()
                }
                frame Disabled {
                }
              }
            }
            frame #2 {
              n201 = Wait (ms)(milliseconds to wait=u32 800) -> ()  [unwired: 1 out]
            }
            frame #3 {
              n202 = disable-structure shown="Enabled" {
                frame Enabled {
                  n203 = while {
                    i -> [w280]
                    stop <- w278 stop-if-true
                    w277 = 0.0 ("Rotation")
                    n204 = Wait (ms)(milliseconds to wait=u32 50) -> ()  [unwired: 1 out]
                    n205 = call <vilib>:"WPI_RobotDriveRefNum Registry Get.vi"("refnum name"="Four Motors") -> ("RobotDriveDevRef"=w283:T13)  [unwired: 1 in, 9 out]
                    n206 = call-poly <vilib>:"WPI_RobotDriveHolonomicDrive.vi"("Rotation"=w277, "Y"=-0.6, "X"=w277, "RobotDriveDevRef"=w283) -> ()  [unwired: 5 in, 3 out]
                    n207 = Greater?(x=w280, y=20) -> (0:w278:bool)
                  }
                  n208 = global write "Robot Global Data.vi" "RC Open"(TRUE ("Enable Vision")) -> ()
                }
                frame Disabled {
                }
              }
            }
            frame #4 {
              n209 = disable-structure shown="Enabled" {
                frame Enabled {
                  w286 = 0.0 ("Rotation")
                  n210 = call <vilib>:"WPI_RobotDriveRefNum Registry Get.vi"("refnum name"="Four Motors") -> ("RobotDriveDevRef"=w288:T13)  [unwired: 1 in, 9 out]
                  n211 = global write "Robot Global Data.vi" "RC Close"(TRUE ("Enable Vision")) -> ()
                  n212 = global write "Robot Global Data.vi" "RC Open"(FALSE ("Enable Vision")) -> ()
                  n213 = call-poly <vilib>:"WPI_RobotDriveHolonomicDrive.vi"("Rotation"=w286, "Y"=w286, "X"=w286, "RobotDriveDevRef"=w288) -> ()  [unwired: 5 in, 3 out]
                }
                frame Disabled {
                }
              }
            }
          }
        }
      }
    }
    frame Disabled {
    }
  }
  "error out" <- w3
  n214 = call-poly <vilib>:"SD Write Value.vi"("Numeric Array"=w10, "Name"="Joystick 0/Axes") -> ()  [unwired: 8 in, 2 out]
